vi "events_for_user.vi"(8 "name_user_option":string, 9 "adres":string, 10 "text_event":string, 11 "size_name":string) -> ()   [LabVIEW 2023]
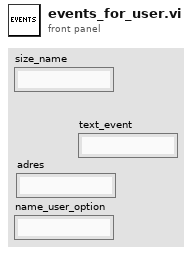
[diagram p1: front panel]
types:
  T1 = enum16{"open", "replace", "create", "open or create", "replace or create", "replace or create with confirmation"}
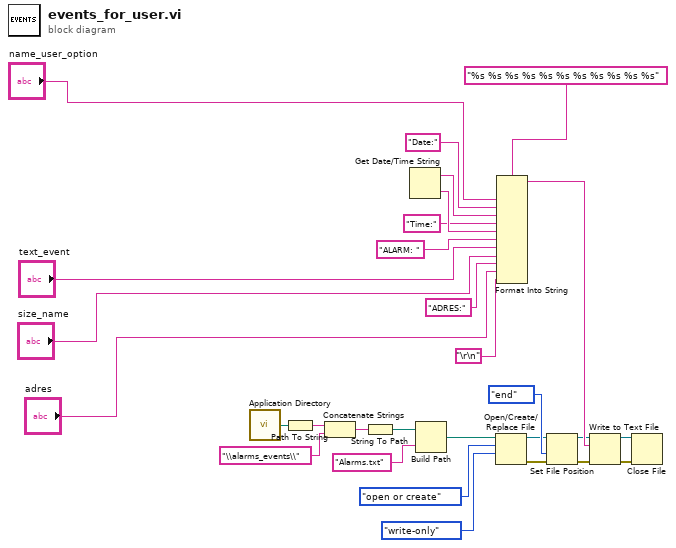
[diagram p0: block diagram]
diagram:
  n1 = call <vilib>:"Application Directory.vi"() -> ("Application Directory"=w23:path)
  n2 = Path To String(path=w23) -> (string=w24:string)
  n3 = Concatenate Strings(w24, "\\alarms_events\\") -> (w26:string)
  n4 = String To Path(string=w26) -> (path=w27:path)
  n5 = Get Date/Time String() -> (date string=w16:string, time string=w18:string)  [unwired: 3 in]
  n6 = Build Path(base path=w27, name or relative path="Alarms.txt") -> (appended path=w28:path)
  n7 = Open/Create/Replace File(file path (use dialog)=w28, operation (0:open)=T1."open or create", access (0:read/write)=enum16{"read/write", "read-only", "write-only"}."write-only") -> (refnum out=w7:refnum<file>, error out=w6:errorcluster)  [unwired: 3 in, 1 out]
  n8 = Format Into String(format string="%s %s %s %s %s %s %s %s %s %s %s", "name_user_option", "Date:" ("format string"), w16, "Time:" ("format string"), w18, "ALARM: " ("format string"), "text_event", "size_name", "ADRES:" ("input 9"), "adres", "\r\n") -> (resulting string=w21:string)  [unwired: 2 in, 1 out]
  n9 = Set File Position(refnum=w7, from (0:start)=enum16{"start", "end", "current"}."end", error in=w6) -> (refnum out=w10:refnum<file>, error out=w11:errorcluster)  [unwired: 1 in]
  n10 = Write to Text File(file (use dialog)=w10, text=w21, error in=w11) -> (refnum out=w9:refnum<file>, error out=w8:errorcluster)  [unwired: 1 in, 1 out]
  n11 = Close File(refnum=w9, error in=w8) -> ()  [unwired: 2 out]
